vi "stroke ratevi.vi"() -> ()   [LabVIEW 2017]
uses:
  <vilib>/measure/NI_MABase.lvlib
panel:
  in  "frequency":dbl=1.0 format="%#_13g"
  out "stroke rate":dbl[](array[numeric])
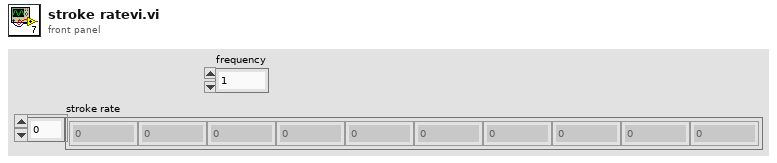
[diagram p1: front panel]
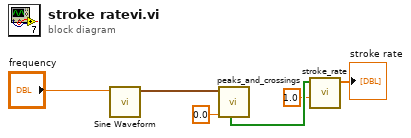
[diagram p0: block diagram]
diagram:
  n1 = call <vilib>:"Sine Waveform.vi"("frequency"="frequency") -> ("signal out"=w3:waveform(dbl))  [unwired: 9 in, 1 out]
  n2 = call "peaks_and_crossings.vi"("crossing level"=0.0, "waveform"=w3) -> ("minus-plus"=w6:bool[])  [unwired: 3 in, 6 out]
  n3 = call "stroke_rate.vi"("dt"=1.0, "minus-plus"=w6) -> ("stroke rate"=→"stroke rate":dbl[])  [unwired: 9 in]
